vi "Parse Response JSON.vi"(8 "error in (no error)":errorcluster, 10 "Response JSON":string, 11 "RGetSceneList in":refnum<class "RGetSceneList.lvclass">) -> (0 "error out":errorcluster, 3 "RGetSceneList out":refnum<class "RGetSceneList.lvclass">)   [LabVIEW 2020, in "obs-websocket.lvlib" / "RGetSceneList.lvclass"]
uses:
  RGetSceneList.lvclass
  RGetSceneList.lvclass/RGetSceneList.ctl
  9ae7c30f-fee4-4b53-a4a1-2e3c8f5f4551.vi
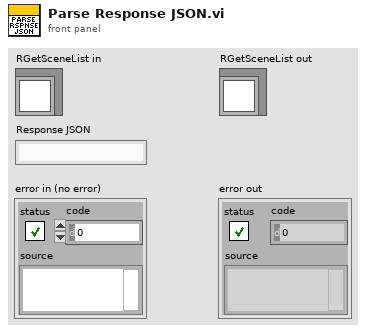
[diagram p1: front panel]
types:
  T1 = cluster{"currentProgramSceneName":string, "currentProgramSceneUuid":string, "currentPreviewSceneName":string, "currentPreviewSceneUuid":string, "scenes":cluster{"sceneIndex":i32, "sceneName":string}[]}
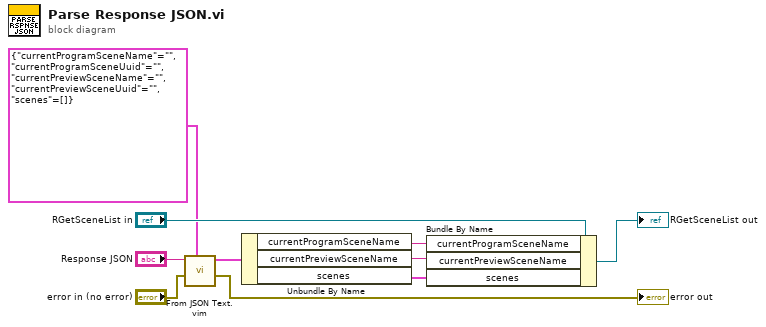
[diagram p0: block diagram]
diagram:
  n1 = call "From JSON Text.vim"("Data Type and Default Value"=T1 {"currentProgramSceneName"="", "currentProgramSceneUuid"="", "currentPreviewSceneName"="", "currentPreviewSceneUuid"="", "scenes"=[]}, "error in (no error)"="error in (no error)", "JSON"="Response JSON") -> ("error out"=→"error out":errorcluster, "Data out"=w6:T1)  [unwired: 7 in]
  n2 = Unbundle By Name(w6) -> ("currentProgramSceneName"=w5:string, "currentPreviewSceneName"=w4:string, "scenes"=w1:cluster{"sceneIndex":i32, "sceneName":string}[])
  n3 = Bundle By Name(cluster="RGetSceneList in", "currentProgramSceneName"=w5, "currentPreviewSceneName"=w4, "scenes"=w1) -> (→"RGetSceneList out":refnum<class "RGetSceneList.lvclass">)
